vi "Get Body Data.vi"(8 "error in (no error)":errorcluster, 11 "Body Reference":refnum<k24>) -> (0 "error out":errorcluster, 3 "BodyData":T1 {"LeanTrackingState" items=["NotTracked", "Inferred", "Tracked"]; "HandRightState" items=["Unknown", "NotTracked", "Open", "Closed", "Lasso"]; "HandRightConfidence" items=["Low", "High"]; "HandLeftState" items=["Unknown", "NotTracked", "Open", "Closed", "Lasso"]; "HandLeftConfidence" items=["Low", "High"]; "ClippedEdges" items=["None"=0, "Right"=1, "Left"=2, "Top"=4, "Bottom"=8]})   [LabVIEW 2014]
uses:
  controls/BodyData.ctl
  Microsoft.Kinect
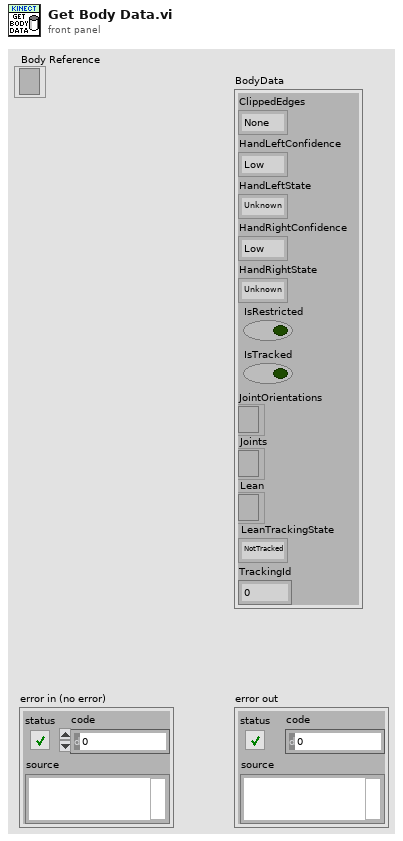
[diagram p1: front panel]
types:
  T1 = typedef "BodyData.ctl" = cluster{"ClippedEdges":i32, "HandLeftConfidence":i32, "HandLeftState":i32, "HandRightConfidence":i32, "HandRightState":i32, "IsRestricted":bool, "IsTracked":bool, "JointOrientations":refnum<k24>, "Joints":refnum<k24>, "Lean":refnum<k24>, "LeanTrackingState":i32, "TrackingId":u64}
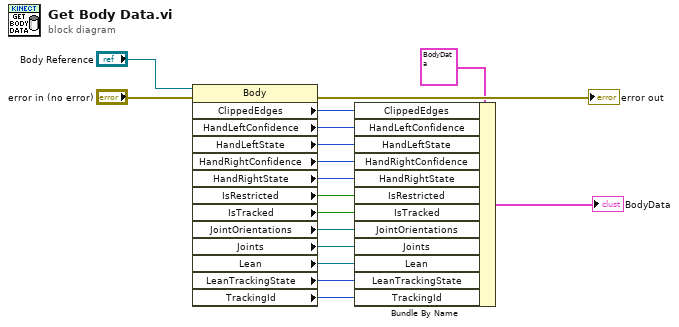
[diagram p0: block diagram]
diagram:
  n1 = property class="Body"(reference="Body Reference", error in="error in (no error)") -> (error out=→"error out":errorcluster, "ClippedEdges"=w13:i32, "HandLeftConfidence"=w12:i32, "HandLeftState"=w11:i32, "HandRightConfidence"=w10:i32, "HandRightState"=w9:i32, "IsRestricted"=w8:bool, "IsTracked"=w7:bool, "JointOrientations"=w6:refnum<k24>, "Joints"=w5:refnum<k24>, "Lean"=w4:refnum<k24>, "LeanTrackingState"=w3:i32, "TrackingId"=w2:u64)  [unwired: 1 out]
  n2 = Bundle By Name(cluster=T1 {"ClippedEdges"=0, "HandLeftConfidence"=0, "HandLeftState"=0, "HandRightConfidence"=0, "HandRightState"=0, "IsRestricted"=FALSE, "IsTracked"=FALSE, "JointOrientations"=refnum, "Joints"=refnum, "Lean"=refnum, "LeanTrackingState"=0, "TrackingId"=0} ("BodyData"), "ClippedEdges"=w13, "HandLeftConfidence"=w12, "HandLeftState"=w11, "HandRightConfidence"=w10, "HandRightState"=w9, "IsRestricted"=w8, "IsTracked"=w7, "JointOrientations"=w6, "Joints"=w5, "Lean"=w4, "LeanTrackingState"=w3, "TrackingId"=w2) -> (→"BodyData":T1)
